vi "Read Histogram Measurements.vi"(0 "VISA resource name":refnum<visa-resource-name>, 11 "error in (no error)":errorcluster) -> (3 "Histogram Peak Hits":i32, 4 "VISA resource name out":refnum<visa-resource-name>, 6 "Histogram Bin Width":dbl, 8 "Histogram Max Bin Hit":dbl, 10 "Histogram Min Bin Hit":dbl, 14 "Histogram Peak-Peak Difference":dbl, 15 "error out":errorcluster)   [LabVIEW 2016, in "Agilent 2000 3000 X-Series.lvlib"]
doc: "Returns basic histogram measurements.\n\n<b>Note:</b>\nThis VI is specific to the 6000-X Series oscilloscopes. These features are not available on other models."
uses:
  Agilent 2000 3000 X-Series.lvlib
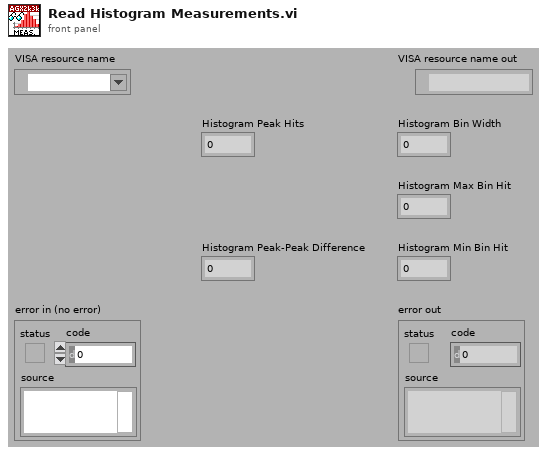
[diagram p1: front panel]
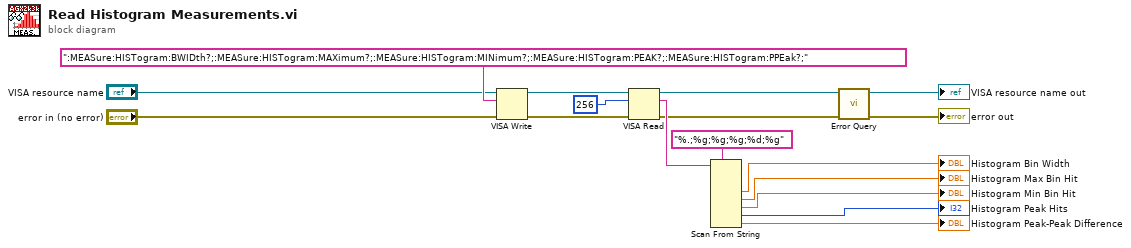
[diagram p0: block diagram]
diagram:
  n1 = VISA Write(VISA resource name="VISA resource name", write buffer=":MEASure:HISTogram:BWIDth?;:MEASure:HISTogram:MAXimum?;:MEASure:HISTogram:MINimum?;:MEASure:HISTogram:PEAK?;:MEASure:HISTogram:PPEak?;", error in (no error)="error in (no error)") -> (VISA resource name out=w13:refnum<visa-resource-name>, error out=w14:errorcluster)  [unwired: 1 out]
  n2 = VISA Read(VISA resource name=w13, byte count=u32 256, error in (no error)=w14) -> (VISA resource name out=w4:refnum<visa-resource-name>, read buffer=w12:string, error out=w3:errorcluster)  [unwired: 1 out]
  n3 = Scan From String(format string="%.;%g;%g;%g;%d;%g", input string=w12) -> (output 1=→"Histogram Bin Width":dbl, output 2=→"Histogram Max Bin Hit":dbl, output 3=→"Histogram Min Bin Hit":dbl, output 4=→"Histogram Peak Hits":i32, output 5=→"Histogram Peak-Peak Difference":dbl)  [unwired: 7 in, 3 out]
  n4 = call "Error Query.vi"("error in (no error)"=w3, "VISA resource name"=w4) -> ("error out"=→"error out":errorcluster, "VISA resource name out"=→"VISA resource name out":refnum<visa-resource-name>)  [unwired: 6 in, 2 out]
